vi "dotNETChart_DisplayChangeEvent.vi"(9 "Chart Settings clstr":T1={"Enable Mouse Zoom (only works in 2D mode)"=TRUE, "Chart Wall Transparency Level"=37, "Chart Wall Colour"=0, "x axis label"="X axis title", "y axis label"="Y axis title", "Enable3D"=TRUE, "3D Settings"={"Inclination"=20, "LightStyle"=2, "Perspective"=4, "WallWidth"=5, "Rotation"=25}, "BackGradientStyle"=2, "SkinStyle"=1, "Chart Background Gradient Colour"=0, "Chart Border Colour"=0, "Palette"=12, "LegendStyle"=0, "ChartType"=[10, 13], "SeriesDataColour"=[]} {"ChartType" items=["Point", "FastPoint", "Bubble", "Line", "Spline", "StepLine", "FastLine", "Bar", "StackedBar", "StackedBar100", "Column", "StackedColumn", "StackedColumn100", "Area", "SplineArea", "StackedArea", "StackedArea100", "Pie", "Doughnut", "Stock", "Candlestick", "Range", "SplineRange", "RangeBar", "RangeColumn", "Radar", "Polar", "ErrorBar", "BoxPlot", "Renko", "ThreeLineBreak", "Kagi", "PointAndFigure", "Funnel", "Pyramid"]; "LegendStyle" items=["Column", "Row", "Table"]; "Palette" items=["None", "Bright", "Grayscale", "Excel", "Light", "Pastel", "EarthTones", "SemiTransparent", "Berry", "Chocolate", "Fire", "SeaGreen", "BrightPastel"]; "SkinStyle" items=["None", "Emboss", "Raised", "Sunken", "FrameThin1", "FrameThin2", "FrameThin3", "FrameThin4", "FrameThin5", "FrameThin6", "FrameTitle1", "FrameTitle2", "FrameTitle3", "FrameTitle4", "FrameTitle5", "FrameTitle6", "FrameTitle7", "FrameTitle8"]; "BackGradientStyle" items=["None", "LeftRight", "TopBottom", "Center", "DiagonalLeft", "DiagonalRight", "HorizontalCenter", "VerticalCenter"]; "3D Settings"."LightStyle" items=["None", "Simplistic", "Realistic"]}, 10 "Microsoft Chart":refnum<k24>) -> (0 "error out":errorcluster, 2 "reference out":refnum<k24>)   [LabVIEW 2013, in "dotNETChart XControl.xctl"]
uses:
  dotNETChart XControl.xctl
  System.Windows.Forms.DataVisualization
  typedefs/ChartSettings cluster.ctl
  typedefs/3DSettings.ctl
  typedefs/BackGradientStyle.ctl
  typedefs/SkinStyle.ctl
  typedefs/Palette.ctl
  typedefs/LegendStyle.ctl
  typedefs/ChartType.ctl
  System.Drawing
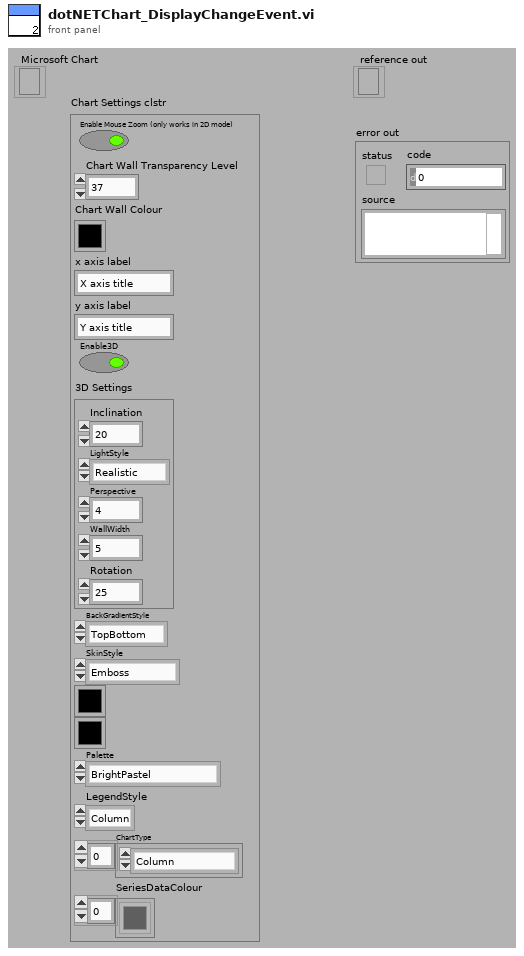
[diagram p1: front panel]
types:
  T1 = typedef "ChartSettings cluster.ctl" = cluster{"Enable Mouse Zoom (only works in 2D mode)":bool, "Chart Wall Transparency Level":i32, "Chart Wall Colour":u32, "x axis label":string, "y axis label":string, "Enable3D":bool, "3D Settings":T2, "BackGradientStyle":T3, "SkinStyle":T4, "Chart Background Gradient Colour":u32, "Chart Border Colour":u32, "Palette":T5, "LegendStyle":T6, "ChartType":T7[], "SeriesDataColour":u32[]}
  T2 = typedef "3DSettings.ctl" = cluster{"Inclination":i32, "LightStyle":i32, "Perspective":i32, "WallWidth":i32, "Rotation":i32}
  T3 = typedef "BackGradientStyle.ctl" = i32
  T4 = typedef "SkinStyle.ctl" = i32
  T5 = typedef "Palette.ctl" = i32
  T6 = typedef "LegendStyle.ctl" = i32
  T7 = typedef "ChartType.ctl" = i32
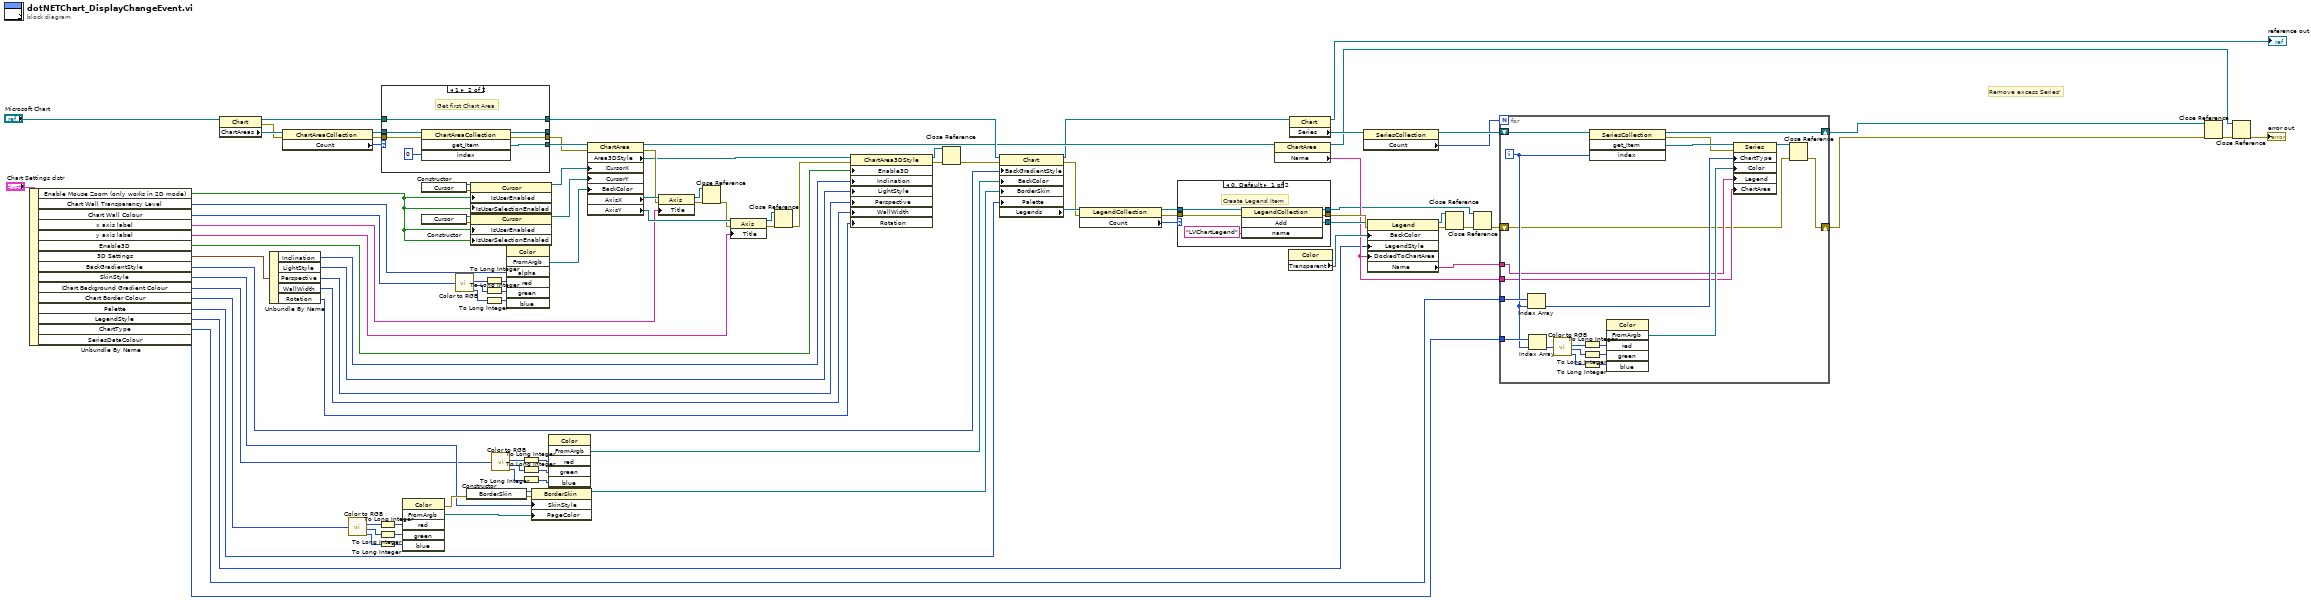
[diagram p0: block diagram]
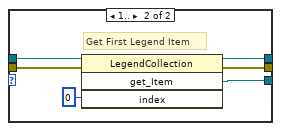
[diagram p2: hidden frame]
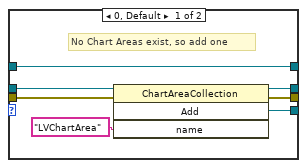
[diagram p3: hidden frame]
diagram:
  # "Remove excess Series'"
  n1 = Unbundle By Name("Chart Settings clstr") -> ("Enable Mouse Zoom (only works in 2D mode)"=w24:bool, "Chart Wall Transparency Level"=w1:i32, "Chart Wall Colour"=w23:u32, "x axis label"=w22:string, "y axis label"=w21:string, "Enable3D"=w20:bool, "3D Settings"=w14:T2, "BackGradientStyle"=w13:T3, "SkinStyle"=w12:T4, "Chart Background Gradient Colour"=w11:u32, "Chart Border Colour"=w10:u32, "Palette"=w9:T5, "LegendStyle"=w8:T6, "ChartType"=w7:T7[], "SeriesDataColour"=w6:u32[])
  n2 = property class="Chart"(reference="Microsoft Chart") -> (reference out=w95:refnum<k24>, error out=w99:errorcluster, "ChartAreas"=w100:refnum<k24>)  [unwired: 1 in]
  n3 = Unbundle By Name(w14) -> ("Inclination"=w19:i32, "LightStyle"=w18:i32, "Perspective"=w17:i32, "WallWidth"=w16:i32, "Rotation"=w15:i32)
  n4 = property class="ChartAreaCollection"(reference=w100, error in=w99) -> (reference out=w97:refnum<k24>, error out=w96:errorcluster, "Count"=w98:i32)
  n5 = call <vilib>:"Color to RGB.vi"("Color"=w10) -> ("R"=w35:u8, "G"=w36:u8, "B"=w37:u8)  [unwired: 1 out]
  n6 = To Long Integer(number=w35) -> (32bit integer=w34:i32)
  n7 = To Long Integer(number=w36) -> (32bit integer=w33:i32)
  n8 = To Long Integer(number=w37) -> (32bit integer=w32:i32)
  n9 = case shown="1" w98 {
    tunnel: w97 -> [w108 w115]
    tunnel: w96 -> [w107 w114]
    tunnel: [w105 w112] -> _
    tunnel: [w104 w111] -> w86
    tunnel: [w103 w110] -> w94
    tunnel: w95 -> [w102 w109]
    tunnel: [w102 w109] -> w68
    frame 0, Default {
      # "No Chart Areas exist, so add one"
      n10 = invoke class="ChartAreaCollection" method="Add"(reference=w108, error in=w107, "name"="LVChartArea") -> (reference out=w105:refnum<k24>, error out=w104:errorcluster, "Add"=w103:refnum<k24>)  [unwired: 1 in, 1 out]
    }
    frame 1 {
      # "Get first Chart Area"
      n11 = invoke class="ChartAreaCollection" method="get_Item"(reference=w115, error in=w114, "index"=0) -> (reference out=w112:refnum<k24>, error out=w111:errorcluster, "get_Item"=w110:refnum<k24>)  [unwired: 1 in, 1 out]
    }
  }
  n12 = invoke class="Color" method="FromArgb"("red"=w34, "green"=w33, "blue"=w32) -> (error out=w81:errorcluster, "FromArgb"=w80:refnum<k24>)  [unwired: 3 in, 4 out]
  n13 = constructor class="Cursor"() -> (reference out=w88:refnum<k24>, error out=w91:errorcluster)  [unwired: 3 in, 1 out]
  n14 = constructor class="Cursor"() -> (reference out=w92:refnum<k24>, error out=w93:errorcluster)  [unwired: 3 in, 1 out]
  n15 = call <vilib>:"Color to RGB.vi"("Color"=w23) -> ("R"=w43:u8, "G"=w42:u8, "B"=w41:u8)  [unwired: 1 out]
  n16 = constructor class="BorderSkin"(error in=w81) -> (reference out=w78:refnum<k24>, error out=w79:errorcluster)  [unwired: 2 in, 1 out]
  n17 = property class="Cursor"(reference=w88, error in=w91, "IsUserEnabled"=w24, "IsUserSelectionEnabled"=w24) -> (reference out=w90:refnum<k24>)  [unwired: 1 out]
  n18 = property class="Cursor"(reference=w92, error in=w93, "IsUserEnabled"=w24, "IsUserSelectionEnabled"=w24) -> (reference out=w89:refnum<k24>)  [unwired: 1 out]
  n19 = To Long Integer(number=w43) -> (32bit integer=w40:i32)
  n20 = To Long Integer(number=w42) -> (32bit integer=w39:i32)
  n21 = To Long Integer(number=w41) -> (32bit integer=w38:i32)
  n22 = call <vilib>:"Color to RGB.vi"("Color"=w11) -> ("R"=w31:u8, "G"=w30:u8, "B"=w29:u8)  [unwired: 1 out]
  n23 = invoke class="Color" method="FromArgb"("alpha"=w1, "red"=w40, "green"=w39, "blue"=w38) -> ("FromArgb"=w2:refnum<k24>)  [unwired: 3 in, 6 out]
  n24 = To Long Integer(number=w31) -> (32bit integer=w28:i32)
  n25 = To Long Integer(number=w30) -> (32bit integer=w27:i32)
  n26 = To Long Integer(number=w29) -> (32bit integer=w26:i32)
  n27 = property class="BorderSkin"(reference=w78, error in=w79, "SkinStyle"=w12, "PageColor"=w80) -> (reference out=w77:refnum<k24>)  [unwired: 1 out]
  n28 = invoke class="Color" method="FromArgb"("red"=w28, "green"=w27, "blue"=w26) -> ("FromArgb"=w82:refnum<k24>)  [unwired: 3 in, 5 out]
  n29 = property class="ChartArea"(reference=w94, error in=w86, "CursorX"=w90, "CursorY"=w89, "BackColor"=w2) -> (reference out=w67:refnum<k24>, error out=w85:errorcluster, "Area3DStyle"=w83:refnum<k24>, "AxisX"=w87:refnum<k24>, "AxisY"=w84:refnum<k24>)
  n30 = property class="Axis"(reference=w87, error in=w85, "Title"=w22) -> (reference out=w58:refnum<k24>, error out=w57:errorcluster)
  n31 = Close Reference(reference=w58, error in (no error)=w57) -> (error out=w56:errorcluster)
  n32 = property class="Axis"(reference=w84, error in=w56, "Title"=w21) -> (reference out=w54:refnum<k24>, error out=w55:errorcluster)
  n33 = Close Reference(reference=w54, error in (no error)=w55) -> (error out=w53:errorcluster)
  n34 = property class="ChartArea3DStyle"(reference=w83, error in=w53, "Enable3D"=w20, "Inclination"=w19, "LightStyle"=w18, "Perspective"=w17, "WallWidth"=w16, "Rotation"=w15) -> (reference out=w59:refnum<k24>, error out=w61:errorcluster)
  n35 = Close Reference(reference=w59, error in (no error)=w61) -> (error out=w60:errorcluster)
  n36 = property class="Chart"(reference=w68, error in=w60, "BackGradientStyle"=w13, "BackColor"=w82, "BorderSkin"=w77, "Palette"=w9) -> (reference out=w66:refnum<k24>, error out=w75:errorcluster, "Legends"=w76:refnum<k24>)
  n37 = property class="LegendCollection"(reference=w76, error in=w75) -> (reference out=w73:refnum<k24>, error out=w72:errorcluster, "Count"=w74:i32)
  n38 = case shown="0, Default" w74 {
    tunnel: w73 -> [w121 w125]
    tunnel: w72 -> [w120 w126]
    tunnel: [w118 w123] -> w70
    tunnel: [w117 w127] -> w71
    tunnel: [w116 w124] -> w48
    frame 0, Default {
      # "Create Legend Item"
      n39 = invoke class="LegendCollection" method="Add"(reference=w121, error in=w120, "name"="LVChartLegend") -> (reference out=w116:refnum<k24>, error out=w117:errorcluster, "Add"=w118:refnum<k24>)  [unwired: 1 in, 1 out]
    }
    frame 1.. {
      # "Get First Legend Item"
      n40 = invoke class="LegendCollection" method="get_Item"(reference=w125, error in=w126, "index"=0) -> (reference out=w124:refnum<k24>, error out=w127:errorcluster, "get_Item"=w123:refnum<k24>)  [unwired: 1 in, 1 out]
    }
  }
  n41 = property class="ChartArea"(reference=w67) -> (reference out=w46:refnum<k24>, "Name"=w63:string)  [unwired: 1 in, 1 out]
  n42 = property class="Color"() -> ("Transparent"=w69:refnum<k24>)  [unwired: 2 in, 2 out]
  n43 = property class="Chart"(reference=w66) -> (reference out=→"reference out":refnum<k24>, "Series"=w65:refnum<k24>)  [unwired: 1 in, 1 out]
  n44 = property class="SeriesCollection"(reference=w65) -> (reference out=w64:refnum<k24>, "Count"=w5:i32)  [unwired: 1 in, 1 out]
  n45 = property class="Legend"(reference=w70, error in=w71, "BackColor"=w69, "LegendStyle"=w8, "DockedToChartArea"=w63) -> (reference out=w51:refnum<k24>, error out=w52:errorcluster, "Name"=w62:string)
  n46 = Close Reference(reference=w51, error in (no error)=w52) -> (error out=w50:errorcluster)
  n47 = Close Reference(reference=w48, error in (no error)=w50) -> (error out=w49:errorcluster)
  n48 = for {
    N: w5 -> [_]
    shift-right: [w129] -> w3
    shift-left: w49 -> [w128]
    shift-right: [w131] -> w4
    shift-left: w64 -> [w148]
    tunnel: w7 -> [w145]
    tunnel: w6 -> [w136]
    tunnel: w63 -> [w132]
    tunnel: w62 -> [w133]
    i -> [w134]
    n49 = Index Array(array=w145, index=w134) -> (element=w144:T7)
    n50 = Index Array(array=w136, index=w134) -> (element=w135:u32)
    n51 = call <vilib>:"Color to RGB.vi"("Color"=w135) -> ("R"=w142:u8, "G"=w141:u8, "B"=w140:u8)  [unwired: 1 out]
    n52 = To Long Integer(number=w142) -> (32bit integer=w139:i32)
    n53 = To Long Integer(number=w141) -> (32bit integer=w138:i32)
    n54 = To Long Integer(number=w140) -> (32bit integer=w137:i32)
    n55 = invoke class="SeriesCollection" method="get_Item"(reference=w148, "index"=w134) -> (reference out=w131:refnum<k24>, error out=w146:errorcluster, "get_Item"=w147:refnum<k24>)  [unwired: 2 in, 1 out]
    n56 = invoke class="Color" method="FromArgb"("red"=w139, "green"=w138, "blue"=w137) -> ("FromArgb"=w143:refnum<k24>)  [unwired: 3 in, 5 out]
    n57 = property class="Series"(reference=w147, error in=w146, "ChartType"=w144, "Color"=w143, "Legend"=w133, "ChartArea"=w132) -> (reference out=w130:refnum<k24>)  [unwired: 1 out]
    n58 = Close Reference(reference=w130, error in (no error)=w128) -> (error out=w129:errorcluster)
  }
  n59 = Close Reference(reference=w4, error in (no error)=w3) -> (error out=w47:errorcluster)
  n60 = Close Reference(reference=w46, error in (no error)=w47) -> (error out=→"error out":errorcluster)
